vi "zadanie_5_plik_tekstowy.vi"() -> ()   [LabVIEW 2024]
uses:
  <vilib>/Utility/file.llb/Write Delimited Spreadsheet (DBL).vi
  <vilib>/Utility/file.llb/Write Delimited Spreadsheet (string).vi
panel:
  out "Read":string
  in  "Select Name":string
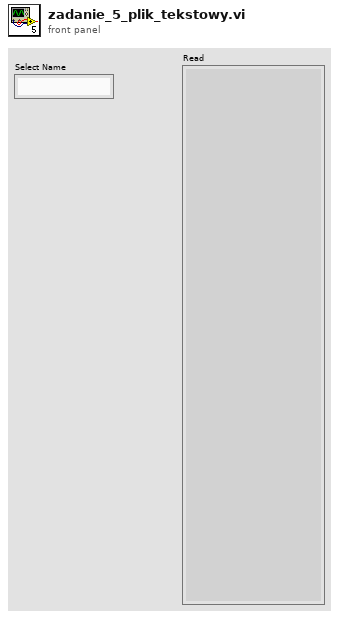
[diagram p1: front panel]
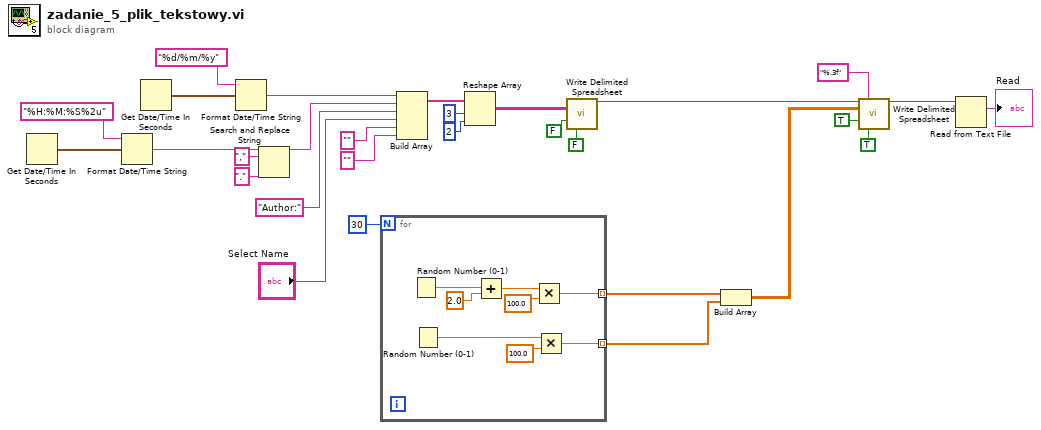
[diagram p0: block diagram]
diagram:
  n1 = Get Date/Time In Seconds() -> (seconds since 1Jan1904=w15:timestamp)
  n2 = Format Date/Time String(time format string (%c)="%H:%M:%S%2u", seconds (now)=w15) -> (date/time string=w14:string)  [unwired: 1 in]
  n3 = Get Date/Time In Seconds() -> (seconds since 1Jan1904=w19:timestamp)
  n4 = Format Date/Time String(time format string (%c)="%d/%m/%y", seconds (now)=w19) -> (date/time string=w18:string)  [unwired: 1 in]
  n5 = Search and Replace String(input string=w14, search string=",", replace string="." ("replace string (\"\")")) -> (result string=w11:string)  [unwired: 5 in, 3 out]
  n6 = for {
    N: 30 -> [_]
    tunnel: [w31] -> w26 mode=indexing
    tunnel: [w30] -> w27 mode=indexing
    n7 = Random Number (0-1)() -> (number: 0 to 1=w37:dbl)
    n8 = Random Number (0-1)() -> (number: 0 to 1=w32:dbl)
    n9 = Add(x=w37, y=2.0) -> (x+y=w35:dbl)
    n10 = Multiply(x=w35, y=100.0) -> (x*y=w30:dbl)
    n11 = Multiply(x=w32, y=100.0) -> (x*y=w31:dbl)
  }
  n12 = Build Array(w18, w11, "Author:" ("element"), "Select Name", "" ("element"), "" ("element")) -> (w10:string[])
  n13 = Reshape Array(w10, 3 ("dimension size"), 2 ("dimension size")) -> (w7:string[][])
  n14 = call-poly <vilib>:"Write Delimited Spreadsheet.vi"("2D data"=w7, "append to file? (new file:F)"=FALSE, "transpose? (no:F)"=FALSE) -> ("new file path (Not A Path if cancelled)"=w20:path)  [unwired: 11 in, 1 out]
  n15 = Build Array(w27, w26) -> (w23:dbl[][])
  n16 = call-poly <vilib>:"Write Delimited Spreadsheet.vi"("file path (dialog if empty)"=w20, "format (%.3f)"="%.3f", "2D data"=w23, "append to file? (new file:F)"=TRUE, "transpose? (no:F)"=TRUE) -> ("new file path (Not A Path if cancelled)"=w1:path)  [unwired: 9 in, 1 out]
  n17 = Read from Text File(file (use dialog)=w1) -> (text=→"Read":string)  [unwired: 3 in, 3 out]
